vi "CMWsub.vi"(8 "error in (no error)":errorcluster, 11 "URL":string="VAC.VGHA_41677/PR") -> (0 "error out":errorcluster, 3 "Numeric":dbl)   [LabVIEW 2014]
uses:
  <userlib>/_RADE/RIO/CMW/classes/CMWSubscribe/openCMWSubscribe.vi
  <userlib>/_RADE/RIO/CMW/classes/CMWSubscribe/CMWSubscribe.vi
  <userlib>/_RADE/RIO/CMW/classes/CMWSubscribe/CMWSubscribe.lvclass
panel:
  out "Data":variant
  out "Loop":i32
  in  "stop":bool
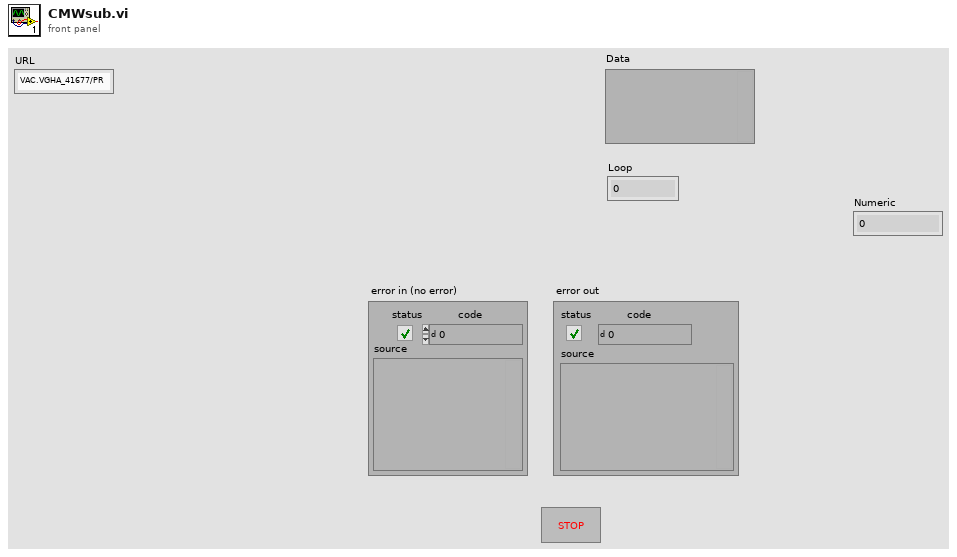
[diagram p1: front panel]
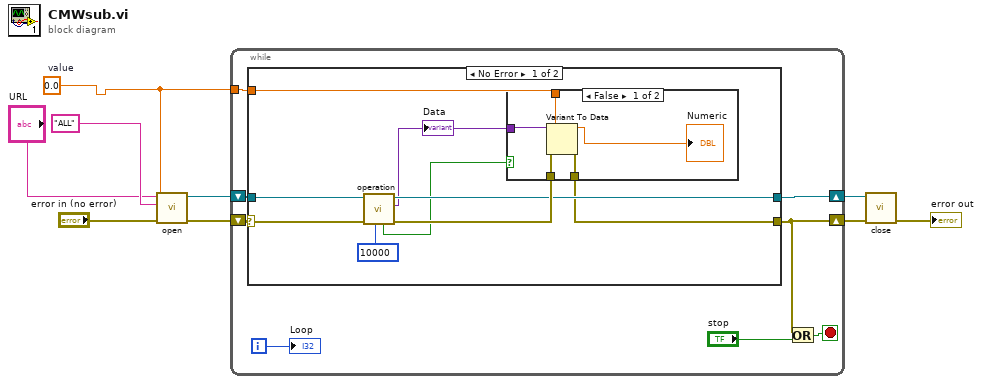
[diagram p0: block diagram]
diagram:
  w1 = sgl 0.0  # value
  n1 = call-poly <userlib>:"open.vi"("error in (no error)"="error in (no error)", "Data type"=w1, "Cycle"="ALL", "URL"="URL") -> ("error out"=w6:errorcluster, "Object out"=w5:refnum<class "CMWSubscribe.lvclass">)  [unwired: 6 in]
  n2 = while {
    shift-right: [w13] -> w4
    shift-left: w6 -> [w17]
    shift-right: [w11] -> w2
    shift-left: w5 -> [w12]
    tunnel: w1 -> [w10]
    i -> [w15]
    stop <- w14 stop-if-true
    n3 = case shown="No Error" w17 {
      selector: w17 -> [w24 w34]
      tunnel: [w22 w34] -> w13
      tunnel: w12 -> [w25 w33]
      tunnel: [w23 w33] -> w11
      tunnel: w10 -> [w21 _]
      frame No Error {
        n4 = call-poly <userlib>:"operation.vi"("Timeout (10000 ms)"=10000, "error in (no error)"=w24, "Object in"=w25) -> ("error out"=w26:errorcluster, "Data"=w20:variant, "Object out"=w23:refnum<class "CMWSubscribe.lvclass">, "Timeout?"=w18:bool)  [unwired: 4 in, 1 out]
        "Data" <- w20
        n5 = case shown="False" w18 {
          tunnel: w26 -> [w31 w32]
          tunnel: [w30 w32] -> w22
          tunnel: w20 -> [w29 _]
          tunnel: w21 -> [w28 _]
          frame False {
            n6 = Variant To Data(error in=w31, type=w28, Variant=w29) -> (data=→"Numeric":sgl, error out=w30:errorcluster)
          }
          frame True {
          }
        }
      }
      frame Error {
      }
    }
    n7 = Or(x=w13, y="stop") -> (x .or. y?=w14:bool)
    "Loop" <- w15
  }
  n8 = call-dynamic "close.vi"("error in (no error)"=w4, "Object in"=w2) -> ("error out"=→"error out":errorcluster)  [unwired: 9 in]
